vi "PH_Watchdog.panel.vi"(0 "object ref":refnum<vi>, 5 "error in (no error)":errorcluster) -> (19 "error out":errorcluster)   [LabVIEW 2014, in "PH_Watchdog.lvlib"]
doc: "By this VI a ross relais can be monitored and switched. \n\nThe indicators \"CLOSED\", \"OPEN\" and \"SWITCH STATE\" show the value of the Beckhoff-Tag: blue indicates bad tag status reference problems, darkgreen false and lightgreen on. If everything is working fine, \"CLOSED\" and \"SWITCH STATE\" should show the same value, while \"OPEN\" has the opposite value. \n\nThe oval button switches the ross relais. It should be in the same state as the \"SWITCH STATE\" indicator. \n\n\"EXIT\" closes the front panel (GUI), while \"Delete Instance\" disconnects and removes the instance from the PCS.\n\nThis VI has no machine safety relevant logig: there is neither a check of internal conclict nor with other objects, for example conflict with other ross relais. Therefore it must be handled with care and should be operated by well educated operators only. It is forseen exclusively for direct operating and testing of the system. \n\nLicense Agreement for this software:\n\nCopyright (C)\nGesellschaft für Schwerionenforschung, GSI\nPlanckstr. 1\n64291 Darmstadt\nGermany\n\nContact: D.Beck@gsi.de \n\nThis program is free software; you can redistribute it and/or modify it under the terms of the GNU General Public License as published by the Free Software Foundation; either version 2 of the license, or (at your option) any later version.\n\nThis program is distributed in the hope that it will be useful, but WITHOUT ANYW ARRANTY; without even the implied warranty of MERCHANTABILITY or FITNESS FOR A PARTICULAR PURPOSE. See the GNU General License for more details (http://www.gnu.org).\n\nGesellschaft für Schwerionenforschung, GSI\nPlanckstr. 1, 64291 Darmstadt, Germany\nFor all questions and ideas contact: M.Richter@gsi.de, H.Brand@gsi.de or D.Beck@gsi.de.\nLast update: 18-DEC-2002"
uses:
  PH_Watchdog.lvlib
  PH_Watchdog.Dataset for GUI.ctl
  PH_Basics/PH_StatusHandler/PH_StatusHandler.GUI element.ctl
  CS_Core/CSObj/CSObj.lvlib
  PH_Basics/PH_Common/PH_Common.lvlib
  PH_Basics/PH_Class/PH_Class.lvlib
  PH_Basics/PH_StatusHandler/PH_StatusHandler.lvlib
panel:
  out "No Info, but linked":string[](array[string])
  out "Alarms":string[](array[string])
  out "Failures":string[](array[string])
  out "All":T1[](array[typedef])
  in  "Delete":bool
  in  "Exit":bool
  # "PCS"
  # "3.40"
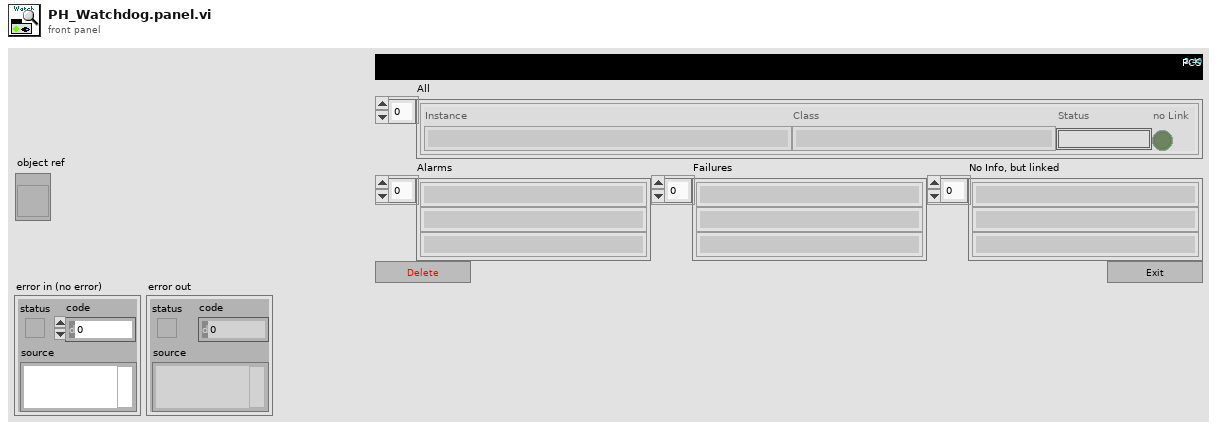
[diagram p1: front panel]
types:
  T1 = typedef "PH_Watchdog.lvlib/PH_Watchdog.Dataset for GUI.ctl" = cluster{"Instance":string, "Class":string, "Status":T2, "no Link":bool}
  T2 = typedef "PH_StatusHandler.lvlib/PH_StatusHandler.GUI element.ctl" = u16
  T3 = typedef "PH_Watchdog.lvlib/PH_Watchdog.i attribute.ctl" = cluster{"GUI Refs":cluster{"All":refnum<vi>, "Failures":refnum<vi>, "Alarms":refnum<vi>, "no info, but linked":refnum<vi>}, "All":T4[]}
  T4 = typedef "PH_Watchdog.lvlib/PH_Watchdog.Dataset.ctl" = cluster{"Instance":string, "Class":string, "Status":T5, "no Link":bool}
  T5 = typedef "PH_StatusHandler.lvlib/PH_StatusHandler.Status.ctl" = i16
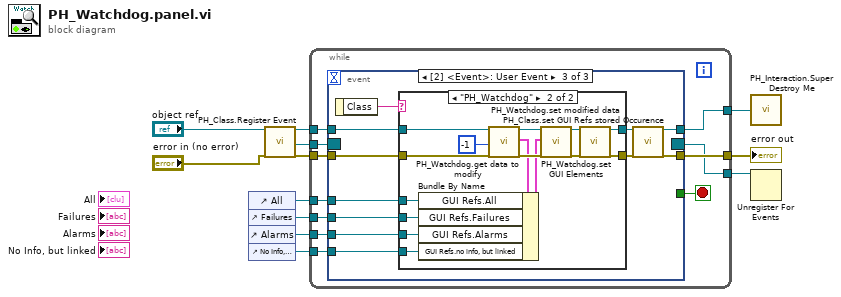
[diagram p0: block diagram]
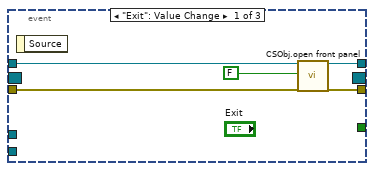
[diagram p2: hidden frame]
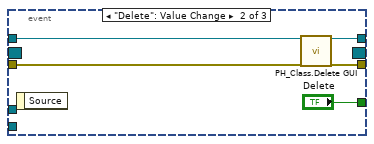
[diagram p3: hidden frame]
diagram:
  n1 = control-ref of="All"() -> (w4:refnum<vi>)
  n2 = control-ref of="Failures"() -> (w3:refnum<vi>)
  n3 = control-ref of="Alarms"() -> (w2:refnum<vi>)
  n4 = control-ref of="No Info, but linked"() -> (w1:refnum<vi>)
  n5 = call "PH_Class.Register Event.vi"("i ref in"="object ref", "error in (no error)"="error in (no error)") -> ("i ref out"=w10:refnum<vi>, "Event Registration Refnum"=w8:refnum<event-registration>, "error out"=w9:errorcluster)  [unwired: 15 in]
  n6 = while {
    tunnel: w10 -> [w20]
    tunnel: [w19] -> w12
    tunnel: w9 -> [w22]
    tunnel: [w21] -> w11
    tunnel: w8 -> [w18]
    tunnel: [w17] -> w7
    tunnel: w4 -> [w16]
    tunnel: w3 -> [w15]
    tunnel: w2 -> [w14]
    tunnel: w1 -> [w13]
    stop <- w23 stop-if-true
    n7 = event shown="[2] <Event>: User Event" {
      selector: w18 -> [_ _ _]
      dyn-events: [_ _ _] -> w17
      timeout: _ -> [_ _ _]
      tunnel: [_ "Delete" _] -> w23
      tunnel: w20 -> [w28 w32 w44]
      tunnel: w22 -> [w26 w31 w41]
      tunnel: [w25 w30 w39] -> w21
      tunnel: [w24 w29 w42] -> w19
      tunnel: w16 -> [_ _ w37]
      tunnel: w15 -> [_ _ w36]
      tunnel: w14 -> [_ _ w35]
      tunnel: w13 -> [_ _ w34]
      event "Exit": Value Change {
        n8 = event-data() -> ()  [unwired: 1 in, 1 out]
        n9 = call "CSObj.open front panel.vi"("i ref in"=w28, "frontPanelOpen"=FALSE ("front panel open"), "error in (no error)"=w26) -> ("i ref out"=w24:refnum<vi>, "error out"=w25:errorcluster)  [unwired: 15 in]
      }
      event "Delete": Value Change {
        n10 = event-data() -> ()  [unwired: 1 in, 1 out]
        n11 = call "PH_Class.Delete GUI.vi"("VI in"=w32, "error in (no error)"=w31) -> ("VI out"=w29:refnum<vi>, "error out"=w30:errorcluster)  [unwired: 16 in]
      }
      event User Event {
        n12 = event-data() -> ("Class"=w38:string)  [unwired: 1 in]
        n13 = case shown="\"PH_Watchdog\"" w38 {
          tunnel: w44 -> [w46 w56]
          tunnel: [w46 w48] -> w43
          tunnel: w41 -> [w45 w55]
          tunnel: [w45 w50] -> w40
          tunnel: w37 -> [_ w53]
          tunnel: w36 -> [_ w52]
          tunnel: w35 -> [_ w51]
          tunnel: w34 -> [_ w47]
          frame Default {
          }
          frame "PH_Watchdog" {
            n14 = call "PH_Watchdog.get data to modify.vi"("i ref in"=w56, "ms timeout (10000)"=-1, "error in (no error)"=w55) -> ("i ref out"=w61:refnum<vi>, "i attribute"=w59:T3, "error out"=w60:errorcluster)  [unwired: 13 in, 1 out]
            n15 = Bundle By Name(cluster=w59, "GUI Refs.All"=w53, "GUI Refs.Failures"=w52, "GUI Refs.Alarms"=w51, "GUI Refs.no info, but linked"=w47) -> (w58:T3)
            n16 = call "PH_Watchdog.set modified data.vi"("i ref in"=w61, "i attribute"=w58, "error in (no error)"=w60) -> ("i ref out"=w49:refnum<vi>, "error out"=w54:errorcluster)  [unwired: 15 in]
            n17 = call "PH_Watchdog.set GUI Elements.vi"("VI in"=w49, "error in"=w54) -> ("VI out"=w48:refnum<vi>, "error out"=w50:errorcluster)  [unwired: 16 in]
          }
        }
        n18 = call "PH_Class.set GUI Refs stored Occurence.vi"("i ref in"=w43, "error in (no error)"=w40) -> ("i ref out"=w42:refnum<vi>, "error out"=w39:errorcluster)  [unwired: 16 in]
      }
    }
  }
  "error out" <- w11
  n19 = call "PH_Interaction.Super Destroy Me.vi"("i ref out"=w12) -> ()
  n20 = Unregister For Events(event registration refnum=w7) -> ()  [unwired: 1 in, 1 out]
